vi "VarifyDataTarget.vi"(8 "error in (no error)":errorcluster, 10 "Destination":string, 11 "DataProcessor in":refnum<class "DataProcessor.lvclass">) -> (0 "error out":errorcluster, 2 "Response?":bool, 3 "DataProcessor out":refnum<class "DataProcessor.lvclass">)   [LabVIEW 2020, in "DataProcessor.lvlib" / "DataProcessor.lvclass"]
uses:
  DataProcessor.lvclass
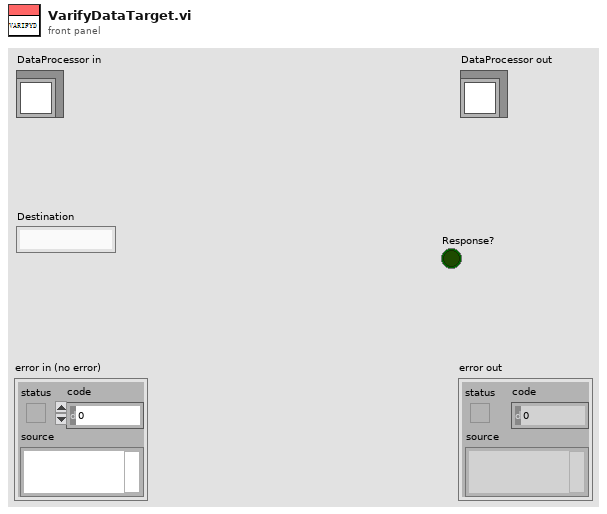
[diagram p1: front panel]
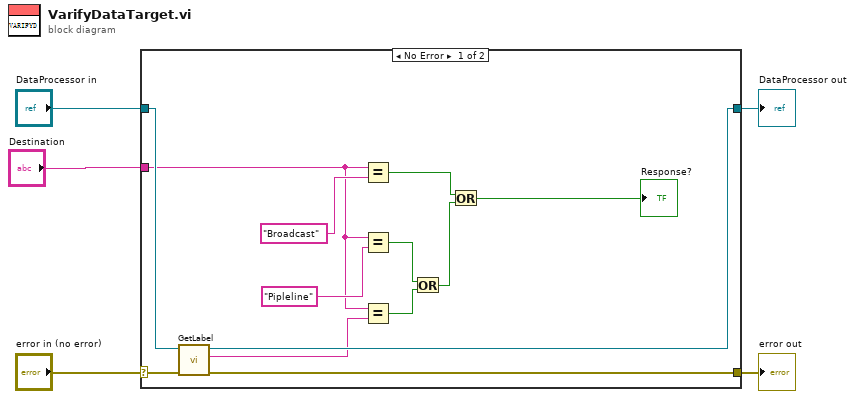
[diagram p0: block diagram]
diagram:
  n1 = case shown="No Error" "error in (no error)" {
    selector: "error in (no error)" -> [w18 w20]
    tunnel: [w10 w20] -> w4
    tunnel: [w8 w19] -> w2
    tunnel: "DataProcessor in" -> [w9 w19]
    tunnel: "Destination" -> [w6 _]
    frame No Error {
      n2 = call-dynamic "GetLabel.vi"("error in (no error)"=w18, "DataProcessor in"=w9) -> ("error out"=w10:errorcluster, "Label"=w7:string, "DataProcessor out"=w8:refnum<class "DataProcessor.lvclass">)  [unwired: 7 in]
      n3 = Equal?(x=w6, y="Broadcast" ("x")) -> (x = y?=w15:bool)
      n4 = Equal?(x=w6, y="Pipleline") -> (x = y?=w14:bool)
      n5 = Equal?(x=w6, y=w7) -> (x = y?=w13:bool)
      n6 = Or(x=w14, y=w13) -> (x .or. y?=w16:bool)
      n7 = Or(x=w15, y=w16) -> (x .or. y?=→"Response?":bool)
    }
    frame Error {
    }
  }
  "error out" <- w4
  "DataProcessor out" <- w2
